vi "HV_Full_Monitor_Single.vi"() -> (3 "Monitor Cluster":T1)   [LabVIEW 2018]
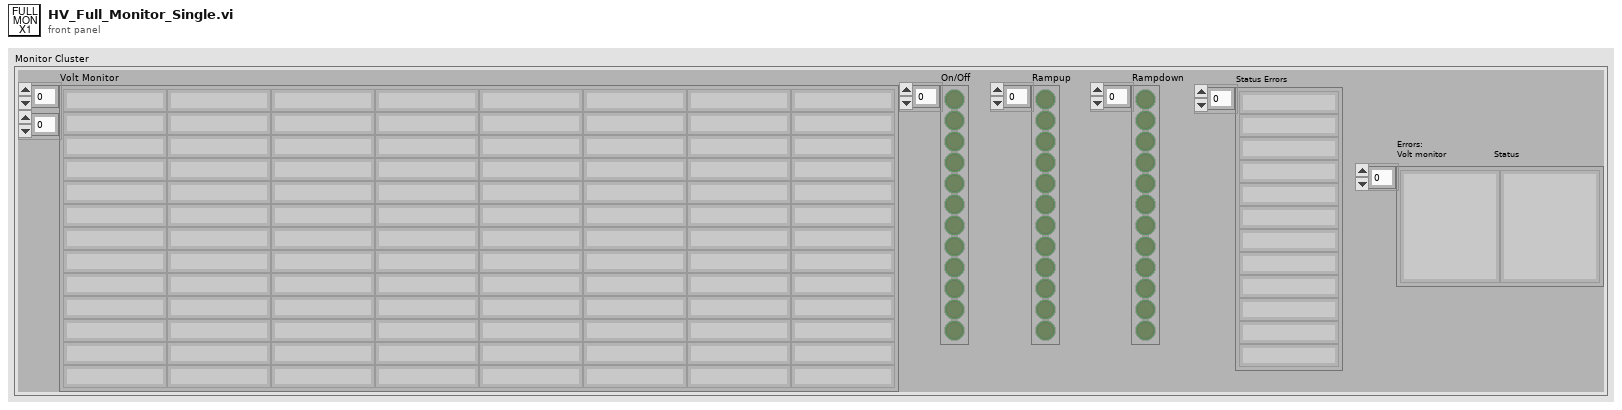
[diagram p1: front panel]
types:
  T1 = cluster{"Volt Monitor":string[][], "On/Off":bool[], "Rampup":bool[], "Rampdown":bool[], "Status Errors":string[], "Errors:\nVolt monitor                Status":string[]}
  T2 = cluster{"Monitor":string[][], "On/Off":bool[], "Rampup":bool[], "Rampdown":bool[], "Status Errors":string[], "Error":string[]}
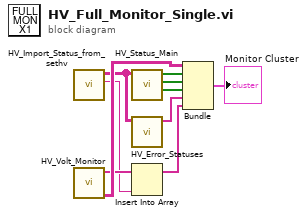
[diagram p0: block diagram]
diagram:
  n1 = call "HV_Import_Status_from_sethv.vi"() -> ("Error"=w3:string, "transposed array"=w5:string[][])  [unwired: 9 in, 1 out]
  n2 = call "HV_Volt_Monitor.vi"() -> ("Monitor"=w6:string[][], "Error"=w4:string[])  [unwired: 10 in]
  n3 = call "HV_Status_Main.vi"("Status Array"=w5) -> ("Rampdown"=w9:bool[], "Rampup"=w8:bool[], "On/Off"=w7:bool[])  [unwired: 8 in]
  n4 = call "HV_Error_Statuses.vi"("transposed array"=w5) -> ("Status Errors"=w10:string[])  [unwired: 10 in]
  n5 = Insert Into Array(array=w4, new element=w3) -> (w2:string[])  [unwired: 1 in]
  n6 = Bundle("Monitor"=w6, "On/Off"=w7, "Rampup"=w8, "Rampdown"=w9, "Status Errors"=w10, "Error"=w2) -> (→"Monitor Cluster":T2)  [unwired: 1 in]
